vi "Microsync set property.vi"(4 "error in (no error)":errorcluster, 5 "VISA resource name":refnum<visa-resource-name>, 10 "Property value":u32, 11 "property":T1(ring)) -> (0 "error out":errorcluster, 3 "VISA resource name out":refnum<visa-resource-name>)   [LabVIEW 2023]
panel:
  in  "Command":string="GET"
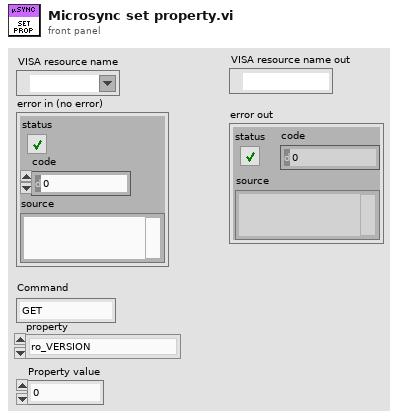
[diagram p1: front panel]
types:
  T1 = enum16{"ro_VERSION", "ro_SYS_TIMER_STATUS", "ro_SYS_TIMER_VALUE", "ro_SYS_TIMER_OVF_COUNT", "ro_SYS_TIME_ms", "ro_SYS_TIMER_PRESCALER", "rw_DFLT_PULSE_DURATION_us", "ro_WATCHDOG_TIMEOUT_ms", "ro_N_EVENTS", "rw_INTLCK_ENABLED", "rw_SELECTED_LASERS", "wo_OPEN_SHUTTERS", "wo_CLOSE_SHUTTERS", "rw_SHUTTER_DELAY_us", "rw_CAM_READOUT_us"}
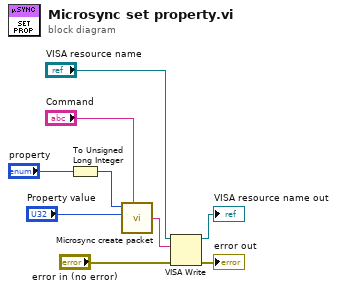
[diagram p0: block diagram]
diagram:
  n1 = To Unsigned Long Integer(number="property") -> (unsigned 32bit integer=w1:u32)
  n2 = call "Microsync create packet.vi"("Command"="Command", "arg2"="Property value", "arg1"=w1) -> ("data packet"=w9:string)  [unwired: 3 in]
  n3 = VISA Write(VISA resource name="VISA resource name", write buffer=w9, error in (no error)="error in (no error)") -> (VISA resource name out=→"VISA resource name out":refnum<visa-resource-name>, error out=→"error out":errorcluster)  [unwired: 1 out]
